vi "Read Roles.vi"(8 "error in (no error)":errorcluster, 11 "5PreparePassGamePlay in":refnum<class "5PreparePassGamePlay.lvclass">) -> (0 "error out":errorcluster, 2 "Roles":T1, 3 "5PreparePassGamePlay out":refnum<class "5PreparePassGamePlay.lvclass">)   [LabVIEW 2021, in "5PreparePassGamePlay.lvclass"]
uses:
  5PreparePassGamePlay.lvclass
  5RobotsRole_class/5RobotsRole.lvclass
  AttackerStopRole_class/AttackerStopRole.lvclass
  5PreparePassGamePlay.lvclass/5PreparePassGamePlay.ctl
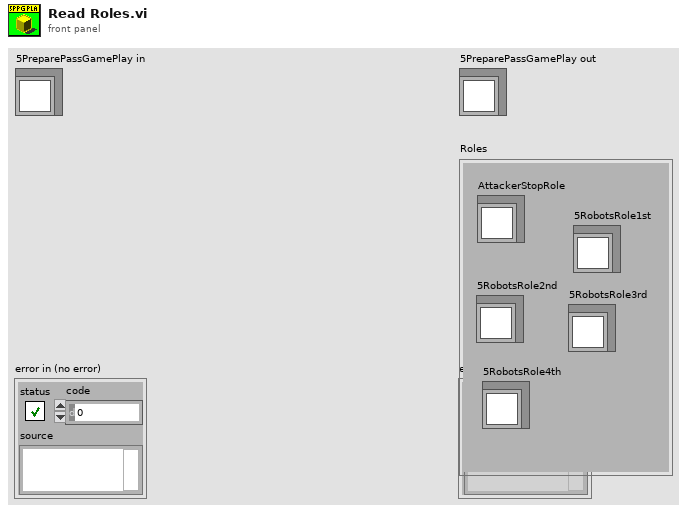
[diagram p1: front panel]
types:
  T1 = cluster{"5RobotsRole1st":refnum<class "5RobotsRole.lvclass">, "5RobotsRole2nd ":refnum<class "5RobotsRole.lvclass">, "5RobotsRole3rd":refnum<class "5RobotsRole.lvclass">, "5RobotsRole4th":refnum<class "5RobotsRole.lvclass">, "AttackerStopRole":refnum<class "AttackerStopRole.lvclass">}
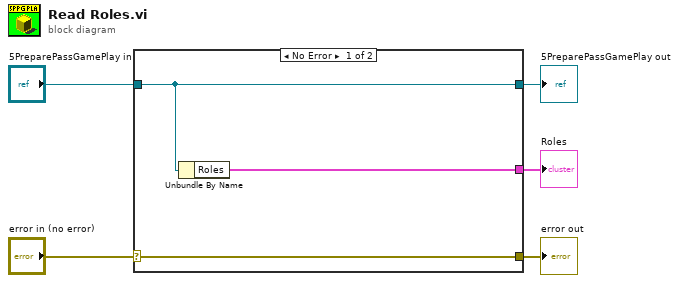
[diagram p0: block diagram]
diagram:
  n1 = case shown="No Error" "error in (no error)" {
    selector: "error in (no error)" -> [w8 w9]
    tunnel: [w8 w9] -> w4
    tunnel: [w7 w10] -> w2
    tunnel: "5PreparePassGamePlay in" -> [w7 w10]
    tunnel: [w6 _] -> w1
    frame No Error {
      n2 = Unbundle By Name(w7) -> ("Roles"=w6:T1)
    }
    frame Error {
    }
  }
  "error out" <- w4
  "5PreparePassGamePlay out" <- w2
  "Roles" <- w1
